vi "Set Result.vi"(8 "error in (no error)":errorcluster, 11 "PostUUT in":refnum<class "PostUUT.lvclass">) -> (0 "error out":errorcluster, 3 "PostUUT out":refnum<class "PostUUT.lvclass">)   [LabVIEW 2019, in "Sequence Main.lvlib" / "PostUUT.lvclass"]
uses:
  PostUUT.lvclass
  PostUUT.lvclass/PostUUT.ctl
  <vilib>/addons/TestStand/_TSUtility.llb/TestStand - Get Property Value (String).vi
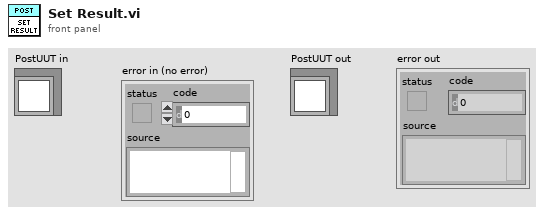
[diagram p1: front panel]
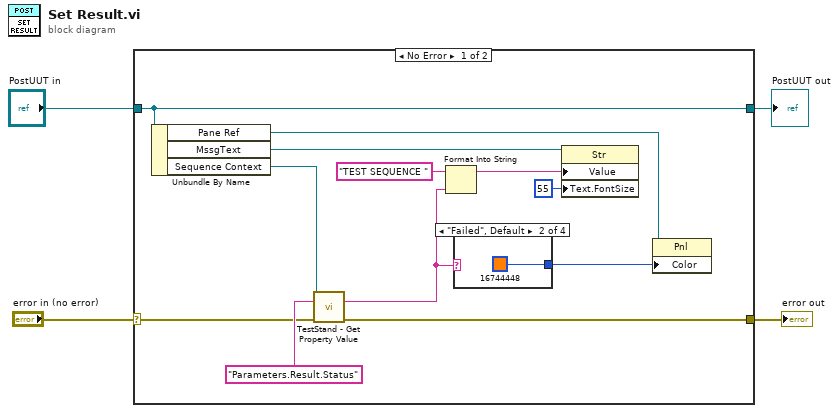
[diagram p0: block diagram]
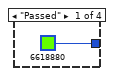
[diagram p2: hidden frame]
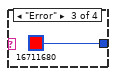
[diagram p3: hidden frame]
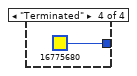
[diagram p4: hidden frame]
diagram:
  n1 = case shown="No Error" "error in (no error)" {
    selector: "error in (no error)" -> [w13 w22]
    tunnel: [w11 w22] -> w3
    tunnel: [w15 w21] -> w1
    tunnel: "PostUUT in" -> [w15 w21]
    frame No Error {
      n2 = Unbundle By Name(w15) -> ("Pane Ref"=w5:refnum<vi>, "MssgText"=w12:refnum<vi>, "Sequence Context"=w14:refnum<k7>)
      n3 = call-poly <vilib>:"TestStand - Get Property Value.vi"("Sequence Context In"=w14, "Lookup String"="Parameters.Result.Status", "error in (no error)"=w13) -> ("Value"=w7:string, "error out"=w11:errorcluster)  [unwired: 10 in, 1 out]
      n4 = Format Into String(initial string="TEST SEQUENCE ", w7) -> (resulting string=w9:string)  [unwired: 2 in, 1 out]
      n5 = case shown="\"Failed\", Default" w7 {
        tunnel: [u32 6618880 ("Color Box") u32 16744448 ("Color Box") u32 16711680 ("Color Box") u32 16775680 ("Color Box")] -> w6
        frame "Passed" {
        }
        frame "Failed", Default {
        }
        frame "Error" {
        }
        frame "Terminated" {
        }
      }
      n6 = property class="Str"(reference=w12, "Value"=w9, "Text.FontSize"=u32 55 ("Text.Font:Size")) -> ()  [unwired: 1 in, 2 out]
      n7 = property class="Pnl"(reference=w5, "Color"=w6) -> ()  [unwired: 1 in, 2 out]
    }
    frame Error {
    }
  }
  "error out" <- w3
  "PostUUT out" <- w1
